vi "Setup_Filepath.vi"(2 "Setup File Type":T1, 3 "Filename in":string) -> (0 "Filename Out":path, 1 "Directory":path)   [LabVIEW 2011]
uses:
  Setup_Filetype.ctl
  Globals/Constants_global.vi
  Globals/Preference_global.vi
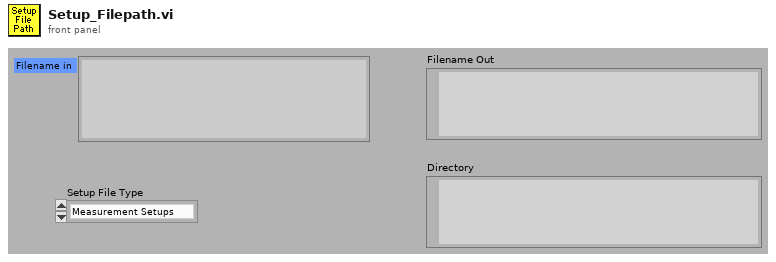
[diagram p1: front panel]
types:
  T1 = typedef "Setup_Filetype.ctl" = enum16{"Measurement Setups", "Calibration Setups", "General", "Results File Plotter Setups", "Speed Calib Tweaks"}
  T2 = typedef "LVDateTimeRec.ctl" = cluster{"fractional second":dbl, "second":i32, "minute":i32, "hour":i32, "day of month":i32, "month":i32, "year":i32, "day of week":i32, "day of year":i32, "DST":i32}
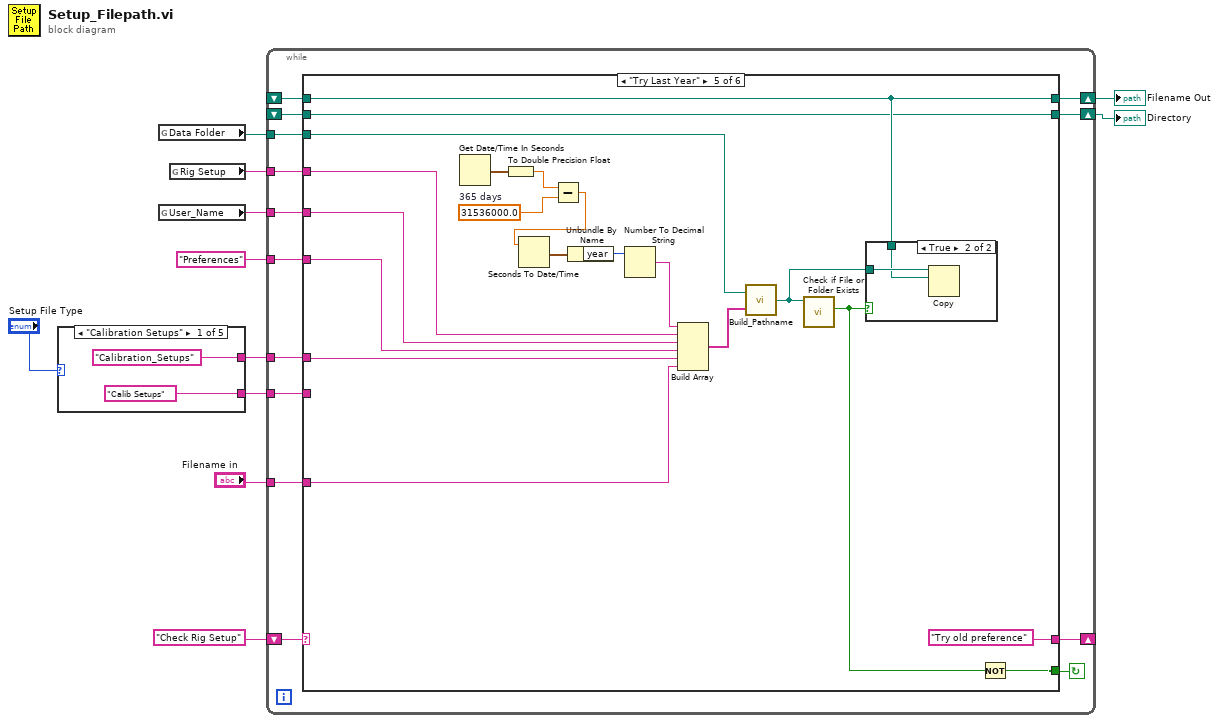
[diagram p0: block diagram]
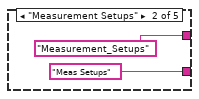
[diagram p2: hidden frame]
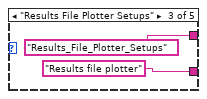
[diagram p3: hidden frame]
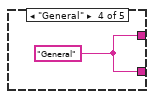
[diagram p4: hidden frame]
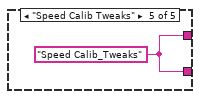
[diagram p5: hidden frame]
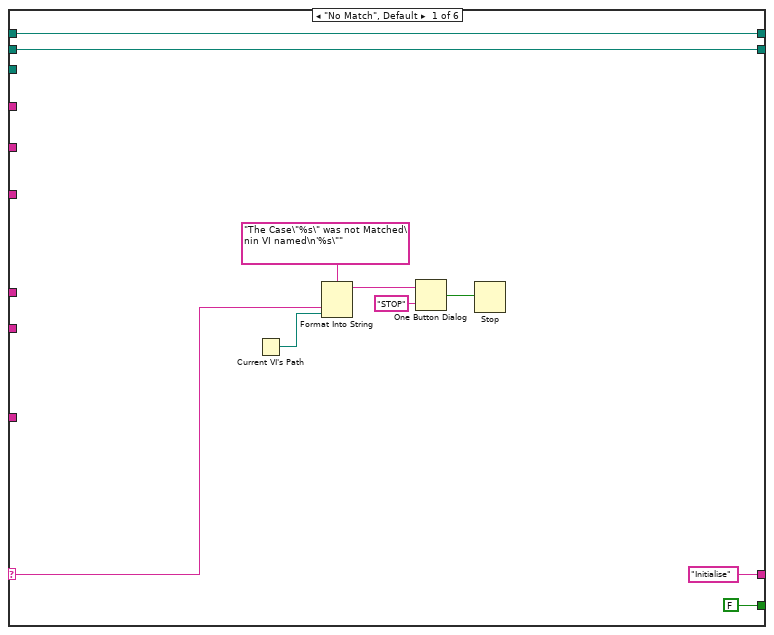
[diagram p6: hidden frame]
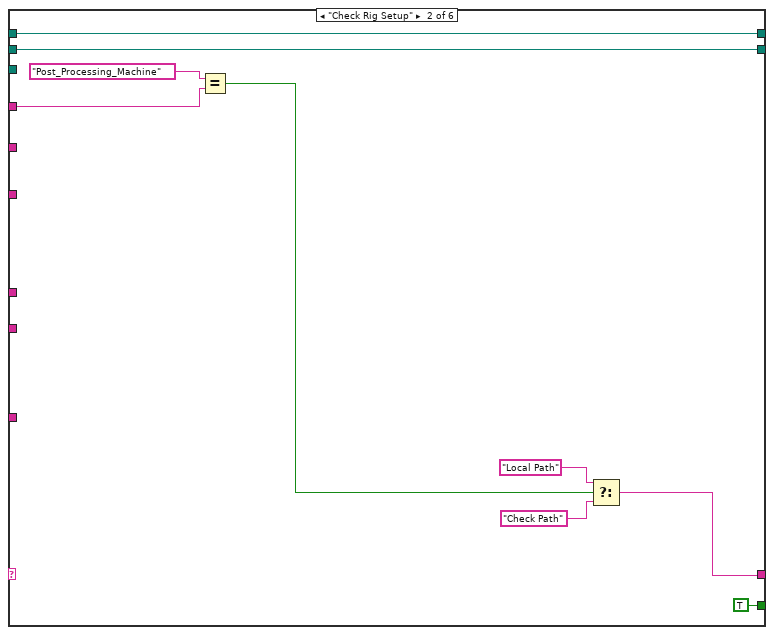
[diagram p7: hidden frame]
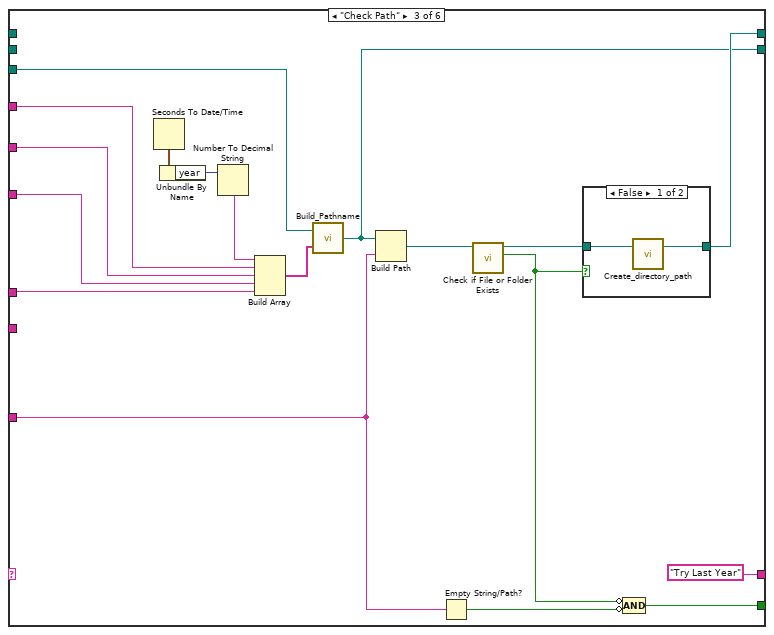
[diagram p8: hidden frame]
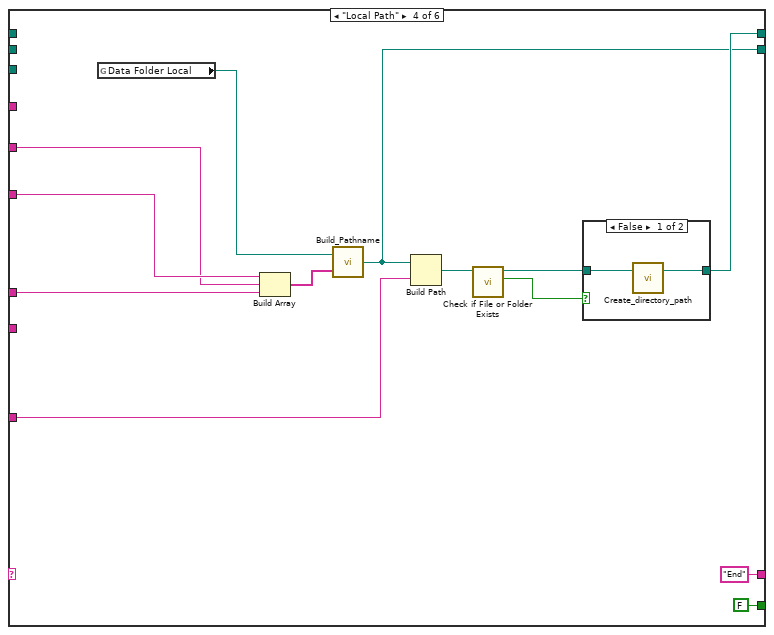
[diagram p10: hidden frame]
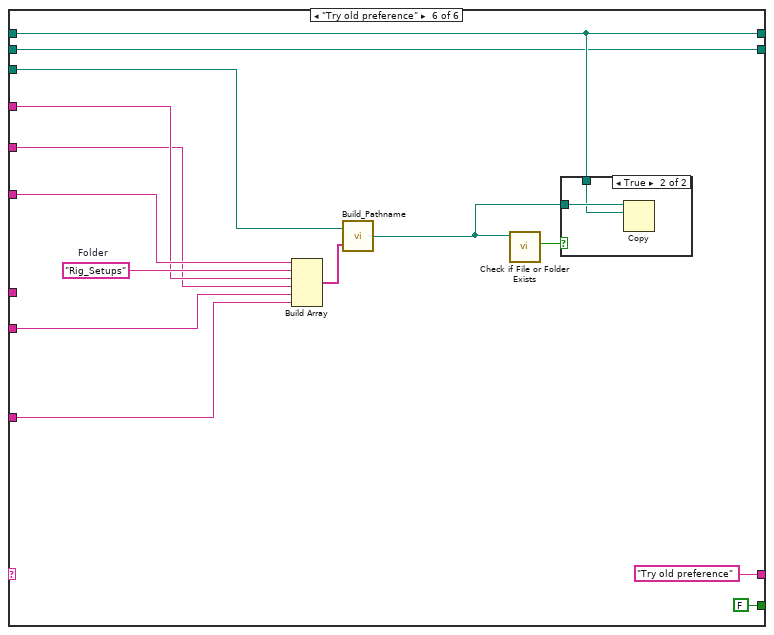
[diagram p13: hidden frame]
diagram:
  n1 = case shown="\"Calibration Setups\"" "Setup File Type" {
    tunnel: ["Calibration_Setups" "Measurement_Setups" "Results_File_Plotter_Setups" w18 w19] -> w3
    tunnel: ["Calib Setups" ("name or relative path") "Meas Setups" ("name or relative path") "Results file plotter" ("name or relative path") w18 w19] -> w2
    frame "Calibration Setups" {
    }
    frame "Measurement Setups" {
    }
    frame "Results File Plotter Setups" {
    }
    frame "General" {
      w18 = "General" ("name or relative path")
    }
    frame "Speed Calib Tweaks" {
      w19 = "Speed Calib_Tweaks" ("name or relative path")
    }
  }
  n2 = global read "Constants_global.vi" "Data Folder"() -> (w10:path)
  n3 = global read "Preference_global.vi" "User_Name"() -> (w8:string)
  n4 = global read "Preference_global.vi" "Rig Setup"() -> (w9:string)
  n5 = while {
    shift-left: "Check Rig Setup" -> [w31]
    shift-right: [w32] -> _
    tunnel: w3 -> [w30]
    tunnel: w10 -> [w29]
    tunnel: w9 -> [w28]
    tunnel: w8 -> [w27]
    tunnel: "Filename in" -> [w26]
    shift-right: [w25] -> w6
    shift-left: _ -> [w24]
    tunnel: "Preferences" ("name or relative path") -> [w23]
    tunnel: w2 -> [w22]
    shift-right: [w21] -> w1
    shift-left: _ -> [w20]
    stop <- w33 continue-if-true
    n6 = case shown="\"Try Last Year\"" w31 {
      selector: w31 -> [w34 _ _ _ _ _]
      tunnel: [FALSE TRUE w58 FALSE w102 FALSE] -> w33
      tunnel: ["Initialise" w45 "Try Last Year" "End" "Try old preference" "Try old preference"] -> w32
      tunnel: w30 -> [_ _ w68 w76 w107 _]
      tunnel: w29 -> [_ _ w67 _ w106 w123]
      tunnel: w28 -> [_ w51 w66 _ w105 w119]
      tunnel: w27 -> [_ _ w65 w77 w104 w118]
      tunnel: w26 -> [_ _ w61 w82 w103 w114]
      tunnel: [w36 w48 w63 w84 w96 w117] -> w25
      tunnel: w24 -> [w36 w48 _ _ w96 w117]
      tunnel: w23 -> [_ _ w57 w78 w95 w121]
      tunnel: w22 -> [_ _ _ _ _ w113]
      tunnel: [w35 w44 w53 w80 w90 w112] -> w21
      tunnel: w20 -> [w35 w44 _ _ w90 w112]
      frame "No Match", Default {
        n7 = Current VI's Path() -> (path=w38:path)
        n8 = Format Into String(format string="The Case\"%s\" was not Matched\nin VI named\n'%s\"" ("Format String"), w34, w38) -> (resulting string=w41:string)  [unwired: 2 in, 1 out]
        n9 = One Button Dialog(message=w41, button name ("OK")="STOP") -> (true=w39:bool)
        n10 = Stop(stop? (T)=w39) -> ()
      }
      frame "Check Rig Setup" {
        n11 = Equal?(x="Post_Processing_Machine" ("Rig Setup"), y=w51) -> (x = y?=w50:bool)
        n12 = Select(t="Local Path", s=w50, f="Check Path") -> (s? t:f=w45:string)
      }
      frame "Check Path" {
        n13 = Seconds To Date/Time() -> (date time rec=w56:T2)  [unwired: 2 out]
        n14 = Unbundle By Name(w56) -> ("year"=w55:i32)
        n15 = Number To Decimal String(number=w55) -> (decimal integer string=w54:string)  [unwired: 1 out]
        n16 = Build Array(w54, w66, w65, w57, w68) -> (w69:string[])
        n17 = call "Build_Pathname.vi"("Output Array"=w69, "Pathname"=w67) -> ("Appended path"=w53:path)
        n18 = Build Path(base path=w53, name or relative path=w61) -> (appended path=w62:path)
        n19 = Empty String/Path?(string/path=w61) -> (empty?=w59:bool)
        n20 = call <vilib>:"Check if File or Folder Exists.vi"("path"=w62) -> ("file or folder exists?"=w60:bool, "dup path"=w64:path)  [unwired: 1 in, 8 out]
        n21 = case shown="False" w60 {
          tunnel: w64 -> [w72 w73]
          tunnel: [w71 w73] -> w63
          frame False {
            n22 = call "Create_directory_path.vi"("Path name"=w72) -> ("Path name Out"=w71:path)  [unwired: 1 in, 1 out]
          }
          frame True {
          }
        }
        n23 = Compound Arithmetic op=AND(invert w60, invert w59) -> (w58:bool)
      }
      frame "Local Path" {
        n24 = global read "Constants_global.vi" "Data Folder Local"() -> (w79:path)
        n25 = Build Array(w78, w77, w76) -> (w86:string[])
        n26 = call "Build_Pathname.vi"("Output Array"=w86, "Pathname"=w79) -> ("Appended path"=w80:path)
        n27 = Build Path(base path=w80, name or relative path=w82) -> (appended path=w83:path)
        n28 = call <vilib>:"Check if File or Folder Exists.vi"("path"=w83) -> ("file or folder exists?"=w81:bool, "dup path"=w85:path)  [unwired: 1 in, 8 out]
        n29 = case shown="False" w81 {
          tunnel: w85 -> [w88 w89]
          tunnel: [w87 w89] -> w84
          frame False {
            n30 = call "Create_directory_path.vi"("Path name"=w88) -> ("Path name Out"=w87:path)  [unwired: 1 in, 1 out]
          }
          frame True {
          }
        }
      }
      frame "Try Last Year" {
        w99 = 31536000.0  # 365 days
        n31 = Get Date/Time In Seconds() -> (seconds since 1Jan1904=w100:timestamp)
        n32 = To Double Precision Float(number=w100) -> (double precision float=w101:dbl)
        n33 = Subtract(x=w101, y=w99) -> (x-y=w92:dbl)
        n34 = Seconds To Date/Time(time stamp (now)=w92) -> (date time rec=w94:T2)  [unwired: 1 out]
        n35 = Unbundle By Name(w94) -> ("year"=w93:i32)
        n36 = Number To Decimal String(number=w93) -> (decimal integer string=w91:string)  [unwired: 1 out]
        n37 = Build Array(w91, w105, w104, w95, w107, w103) -> (w108:string[])
        n38 = call "Build_Pathname.vi"("Output Array"=w108, "Pathname"=w106) -> ("Appended path"=w98:path)
        n39 = call <vilib>:"Check if File or Folder Exists.vi"("path"=w98) -> ("file or folder exists?"=w97:bool)  [unwired: 1 in, 9 out]
        n40 = case shown="True" w97 {
          tunnel: w98 -> [_ w111]
          tunnel: w96 -> [_ w110]
          frame False {
          }
          frame True {
            n41 = Copy(10:w110, 11:w111) -> ()  [unwired: 3 in, 3 out]
          }
        }
        n42 = Not(x=w97) -> (.not. x?=w102:bool)
      }
      frame "Try old preference" {
        w120 = "Rig_Setups"  # Folder
        n43 = Build Array(w121, w120, w119, w118, w113, w114) -> (w124:string[])
        n44 = call "Build_Pathname.vi"("Output Array"=w124, "Pathname"=w123) -> ("Appended path"=w115:path)
        n45 = call <vilib>:"Check if File or Folder Exists.vi"("path"=w115) -> ("file or folder exists?"=w122:bool)  [unwired: 1 in, 9 out]
        n46 = case shown="True" w122 {
          tunnel: w115 -> [_ w127]
          tunnel: w117 -> [_ w126]
          frame False {
          }
          frame True {
            n47 = Copy(10:w126, 11:w127) -> ()  [unwired: 3 in, 3 out]
          }
        }
      }
    }
  }
  "Filename Out" <- w6
  "Directory" <- w1
